vi "Line2001.vi"   [LabVIEW 2013]
uses:
  <vilib>/Heliosphere Research LLC/Advanced Plotting Toolkit/Advanced Plotting Toolkit.lvlib
types:
  T1 = typedef "Advanced Plotting Toolkit.lvlib/PlotID.ctl" = i32
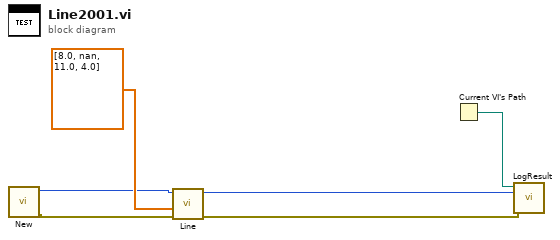
[diagram p0: block diagram]
diagram:
  n1 = call <vilib>:"New.vi"() -> ("error out"=w2:errorcluster, "Plot ID"=w4:T1)  [unwired: 10 in]
  n2 = call <vilib>:"Line.vi"("error in (no error)"=w2, "Y Data"=dbl[] [8.0, nan, 11.0, 4.0], "Plot ID"=w4) -> ("error out"=w1:errorcluster, "Plot ID out"=w3:T1)  [unwired: 7 in]
  n3 = Current VI's Path() -> (path=w6:path)
  n4 = call "LogResult.vi"("Test Result"=w1, "Test Artifact"=w3, "VI Path"=w6) -> ()  [unwired: 9 in]
